vi "findV0.vi"(7 "array":dbl[][](array[numeric]), 8 "error in (no error)":errorcluster, 9 "delta":dbl, 10 "est_vel":dbl, 11 "Game in":refnum<class "Game.lvclass">) -> (0 "error out":errorcluster, 2 "appended array":dbl[][](array[numeric]), 3 "Game out":refnum<class "Game.lvclass">)   [LabVIEW 2023, in "Game.lvclass"]
uses:
  Game.lvclass
  efcc8cff-0d10-40f9-bdb3-533c7b50b309.vi
  <vilib>/Array/Sort 2D Array - Pop Stack.vi
  <vilib>/Array/Sort 2D Array - Push Stack.vi
  efcc8cff-0d10-40f9-bdb3-533c7b50b309.vi/269d4b3b-47f5-49e3-8884-44851e4dd9d5.vi
  efcc8cff-0d10-40f9-bdb3-533c7b50b309.vi/6d99389c-673d-4efb-bf33-19b32bcf4cf8.vi
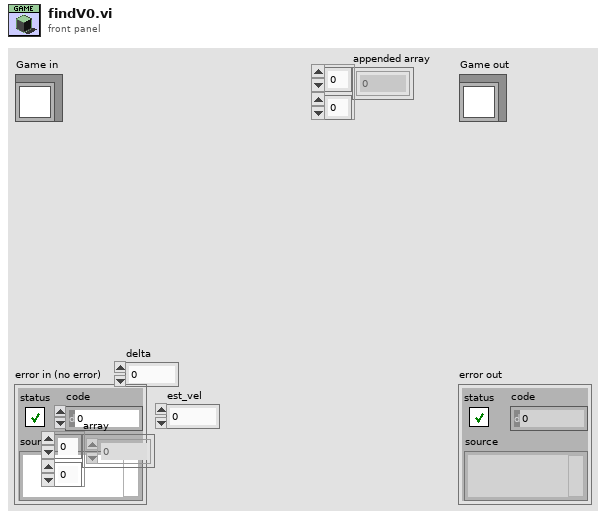
[diagram p1: front panel]
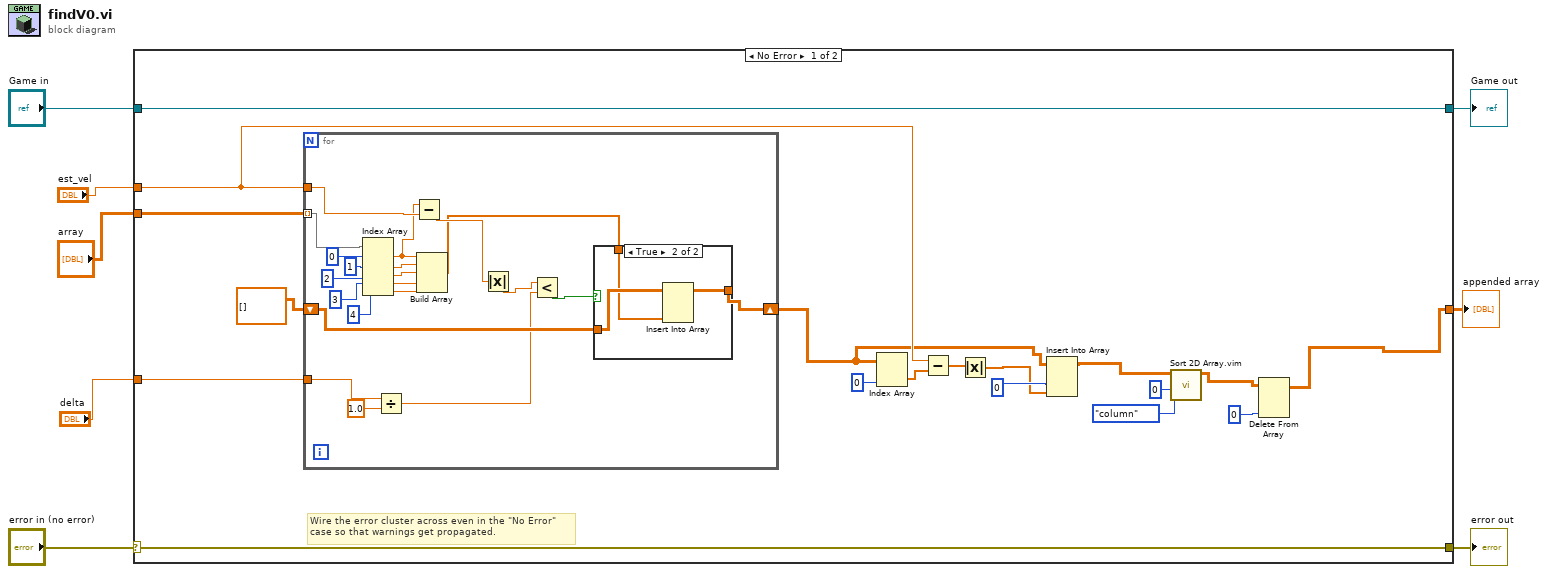
[diagram p0: block diagram]
diagram:
  n1 = case shown="No Error" "error in (no error)" {
    selector: "error in (no error)" -> [w25 w53]
    tunnel: [w25 w53] -> w7
    tunnel: [w26 w52] -> w5
    tunnel: "Game in" -> [w26 w52]
    tunnel: "est_vel" -> [w17 _]
    tunnel: "array" -> [w23 _]
    tunnel: "delta" -> [w22 _]
    tunnel: [w9 _] -> w1
    frame No Error {
      # "Wire the error cluster across even in the \"No Error\"\ncase so that warnings get propagated."
      n2 = for {
        tunnel: w23 -> [w47] mode=indexing
        tunnel: w17 -> [w44]
        tunnel: w22 -> [w35]
        shift-right: [w36] -> w16
        shift-left: dbl[][] [] ("appended array") -> [w40]
        n3 = Index Array(array=w47, index #1=0 ("index"), index #2=1 ("index"), index #3=2 ("index"), index #4=3 ("index"), index #5=4 ("index")) -> (element #1=w31:dbl, element #2=w38:dbl, element #3=w39:dbl, element #4=w28:dbl, element #5=w27:dbl)
        n4 = Divide(x=w35, y=1.0) -> (x/y=w33:dbl)
        n5 = Subtract(x=w31, y=w44) -> (x-y=w43:dbl)
        n6 = Build Array(w31, w38, w39, w28, w27) -> (w37:dbl[])
        n7 = Absolute Value(x=w43) -> (abs(x)=w42:dbl)
        n8 = Less?(x=w42, y=w33) -> (x < y?=w41:bool)
        n9 = case shown="True" w41 {
          tunnel: w40 -> [w48 w51]
          tunnel: w37 -> [_ w50]
          tunnel: [w48 w49] -> w36
          frame False {
          }
          frame True {
            n10 = Insert Into Array(array=w51, new element=w50) -> (w49:dbl[][])  [unwired: 2 in]
          }
        }
      }
      n11 = Index Array(array=w16, index (col)=0 ("disabled index (col)")) -> (element=w12:dbl[])  [unwired: 1 in]
      n12 = Subtract(x=w17, y=w12) -> (x-y=w20:dbl[])
      n13 = Absolute Value(x=w20) -> (abs(x)=w14:dbl[])
      n14 = Insert Into Array(array=w16, index (col)=0 ("disabled index (col)"), new element=w14) -> (w13:dbl[][])  [unwired: 1 in]
      n15 = call "Sort 2D Array.vim"("index"=0, "dimension to index (column)"=enum16{"column", "row"}."column", "2D array"=w13) -> ("sorted 2D array"=w11:dbl[][])  [unwired: 7 in, 1 out]
      n16 = Delete From Array(array=w11, index (col)=0 ("disabled index (col)")) -> (array with subset deleted=w9:dbl[][])  [unwired: 2 in, 1 out]
    }
    frame Error {
    }
  }
  "error out" <- w7
  "Game out" <- w5
  "appended array" <- w1
